vi "plot_missions.vi"(9 "MapDistanceInfo":T1 {"Top Left Pixel UTM"."North" format="%#_10f"; "Top Left Pixel UTM"."East" format="%#_8f"; "Bottom Right Pixel UTM"."North" format="%#_10f"; "Bottom Right Pixel UTM"."East" format="%#_8f"}, 10 "Missions":refnum<class "GenericMission.lvclass">[](array[class]), 11 "Map in":T3) -> (1 "MapDistanceInfo OUT":T1 {"Top Left Pixel UTM"."North" format="%#_10f"; "Top Left Pixel UTM"."East" format="%#_8f"; "Bottom Right Pixel UTM"."North" format="%#_10f"; "Bottom Right Pixel UTM"."East" format="%#_8f"}, 2 "WP Outside Img":bool, 3 "Map Out":T3)   [LabVIEW 2013]
doc: "Takes in a list of missions, extracts the key coordinates, turns them into waypoints, and plots them."
uses:
  cRIO_Code/Logic/Classes/Waypoint/Waypoint.lvclass
  <vilib>/vision/Image Controls.llb/IMAQ Image.ctl
  TypeDef/map_metadata.ctl
  cRIO_Code/Data/TypeDefs/UTM Location.ctl
  cRIO_Code/Logic/Classes/Missions/GenericMission/GenericMission.lvclass
panel:
  out "Waypoint Array":refnum<class "Waypoint.lvclass">[](array[class])
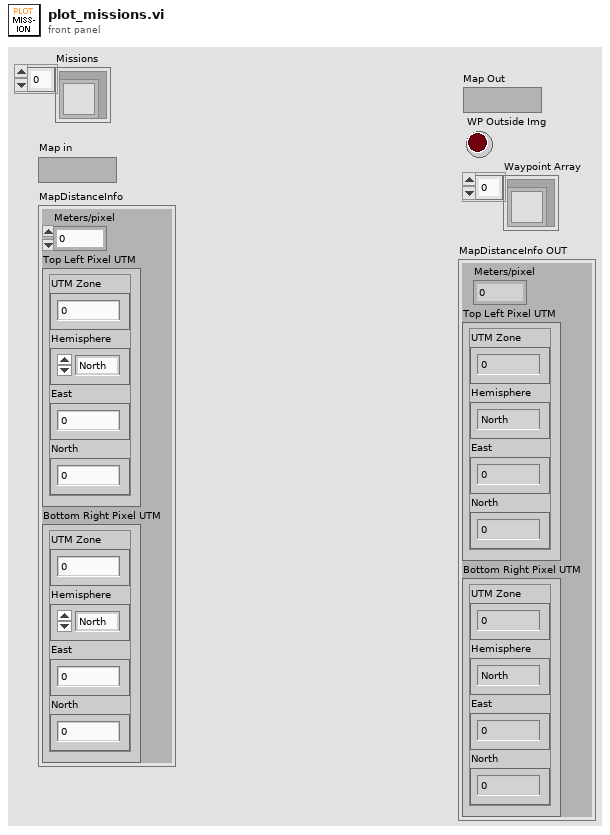
[diagram p1: front panel]
types:
  T1 = typedef "map_metadata.ctl" = cluster{"Meters/pixel":dbl, "Top Left Pixel UTM":T2, "Bottom Right Pixel UTM":T2}
  T2 = typedef "UTM Location.ctl" = cluster{"UTM Zone":dbl, "Hemisphere":enum16{"North", "South"}, "East":dbl, "North":dbl}
  T3 = typedef "IMAQ Image.ctl" = refnum<image>
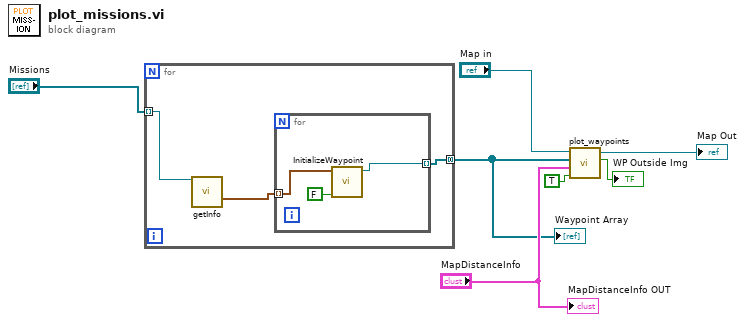
[diagram p0: block diagram]
diagram:
  n1 = for {
    tunnel: "Missions" -> [w10] mode=indexing
    tunnel: [w8] -> w1 mode=concatenating
    n2 = call-dynamic "getInfo.vi"("GenericMission in"=w10) -> ("Points of Interest"=w9:T2[])  [unwired: 6 in, 8 out]
    n3 = for {
      tunnel: w9 -> [w13] mode=indexing
      tunnel: [w11] -> w8 mode=indexing
      n4 = call "InitializeWaypoint.vi"("Sailing Point?"=FALSE, "Coords"=w13) -> ("Waypoint Out"=w11:refnum<class "Waypoint.lvclass">)  [unwired: 9 in]
    }
  }
  "Waypoint Array" <- w1
  n5 = call "plot_waypoints.vi"("Mission Waypoint?"=TRUE, "MapDistanceInfo"="MapDistanceInfo", "Waypoint Array"=w1, "Map in"="Map in") -> ("WP Outside Img"=→"WP Outside Img":bool, "Map Out"=→"Map Out":T3)  [unwired: 6 in]
  "MapDistanceInfo OUT" <- "MapDistanceInfo"
